vi "test.vi"   [LabVIEW 2022 SP3]
uses:
  LV_ScreenCapture.dll
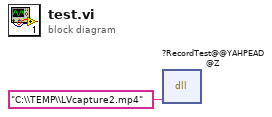
[diagram p0: block diagram]
diagram:
  n1 = dll-call lib="C:/Users/Andrey/Documents/GitHub/ScreenCaptureDirectX/x64/Release/LV_ScreenCapture.dll" fn="?RecordTest@@YAHPEAD@Z"("path"="C:\\TEMP\\LVcapture2.mp4") -> ()  [unwired: 5 in, 2 out]
